vi "FG Set Standard State.vi"(8 "error in (no error)":errorcluster, 9 "voltage (Vpp)":dbl[unit], 10 "Channel (0: Channel 1)":T1 items=["Channel 1", "Channel 2"], 11 "VISA resource name":refnum<visa-resource-name>) -> (0 "error out":errorcluster, 3 "VISA resource name out":refnum<visa-resource-name>)   [LabVIEW 2009]
uses:
  Tektronix AFG 3000 Series/controls.llb/Channel.ctl
  Tektronix AFG 3000 Series/controls.llb/Frequency Mode.ctl
  Tektronix AFG 3000 Series/controls.llb/Waveform Shape.ctl
  Tektronix AFG 3000 Series/controls.llb/Volt Unit.ctl
  Tektronix AFG 3000 Series/controls.llb/Voltage.ctl
  Tektronix AFG 3000 Series/Tektronix AFG 3000 Series.lvlib
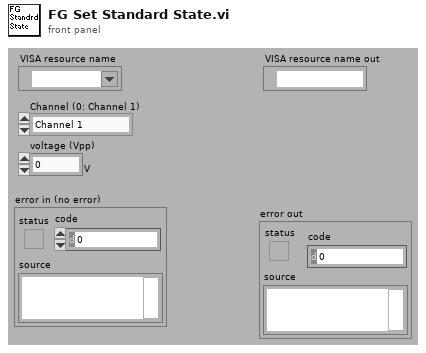
[diagram p1: front panel]
types:
  T1 = typedef "Channel.ctl" = u16
  T2 = typedef "Voltage.ctl" = enum16{"amplitude", "offset", "high", "low", "high limit", "low limit"}
  T3 = typedef "Volt Unit.ctl" = enum16{"VPP", "VRMS", "DBM"}
  T4 = typedef "Waveform Shape.ctl" = u16
  T5 = typedef "Frequency Mode.ctl" = enum16{"CW", "Sweep"}
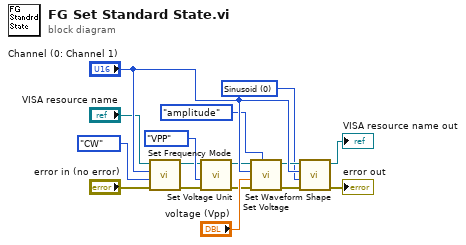
[diagram p0: block diagram]
diagram:
  w11 = T4 0 items=["Sinusoid", "Square", "Pulse", "Ramp", "PRNoise", "DC", "SINC", "Gaussian", "Lorentz", "ERise", "EDecay", "Haversine", "User 1", "User 2", "User 3", "User 4", "EMemory", "EFile"] ("Waveform Shape")
  n1 = call "Set Frequency Mode.vi"("error in (no error)"="error in (no error)", "Mode (0: CW)"=Frequency_Mode."CW", "Channel (0: Channel 1)"="Channel (0: Channel 1)", "VISA resource name"="VISA resource name") -> ("error out"=w4:errorcluster, "VISA resource name out"=w6:refnum<visa-resource-name>)  [unwired: 6 out]
  n2 = call "Set Voltage Unit.vi"("error in (no error)"=w4, "Volt Unit (VPP)"=Volt_Unit."VPP", "VISA resource name"=w6) -> ("error out"=w3:errorcluster, "VISA resource name out"=w5:refnum<visa-resource-name>)  [unwired: 1 in, 6 out]
  n3 = call "Set Voltage.vi"("Voltage Param (amplitude)"=Voltage."amplitude", "error in (no error)"=w3, "voltage"="voltage (Vpp)", "Channel (0: Channel 1)"="Channel (0: Channel 1)", "VISA resource name"=w5) -> ("error out"=w14:errorcluster, "VISA resource name out"=w15:refnum<visa-resource-name>)  [unwired: 5 out]
  n4 = call "Set Waveform Shape.vi"("error in (no error)"=w14, "Waveform Shape"=w11, "Channel (0: Channel 1)"="Channel (0: Channel 1)", "VISA resource name"=w15) -> ("error out"=→"error out":errorcluster, "VISA resource name out"=→"VISA resource name out":refnum<visa-resource-name>)  [unwired: 6 out]
